vi "Simulation.vi"() -> ()   [LabVIEW 2025]
uses:
  <vilib>/Platform/TimedLoop/XDataNode/timing_clust.ctl
  <vilib>/Platform/TimedLoop/XDataNode/nitl_modes.ctl
  <vilib>/Platform/TimedLoop/XDataNode/wakeup.ctl
  <vilib>/Analysis/5stat.llb/RMS (DBL).vi
  <vilib>/platform/TimedLoop/XDataNode/XDataNode.xnode
  <vilib>/Platform/TimedLoop/XDataNode/XDNodeRunTimeDep.lvlib
  <vilib>/Analysis/NI_AALBase.lvlib
  <vilib>/ptbypt/NI_PtbyPt.lvlib
  <vilib>/Analysis/NI_AALPro.lvlib
panel:
  in  "stop":bool
  out "CLoop":i32
  out "TCP loop":i32
  out "velocity":dbl[](graph)
  out "rms error":dbl format="%0.2f"
  out "TCP":errorcluster
  out "Error":string
  out "Done 2":bool caption="TCP Done"
  out "Path":dbl[](graph)
  out "Output":dbl[](graph)
  out "Error":dbl[](graph)
  out "限制上限":bool
  out "Delay":i32
  out "Done":bool caption="Run Done"
  in  "停止":bool
  in  "開始執行":bool
  out "data length":i32
  out "pdl":i32
  out "Total time":i32
  out "Ts":dbl=0.001
  in  "初始化":bool
  # "資料儲存區"
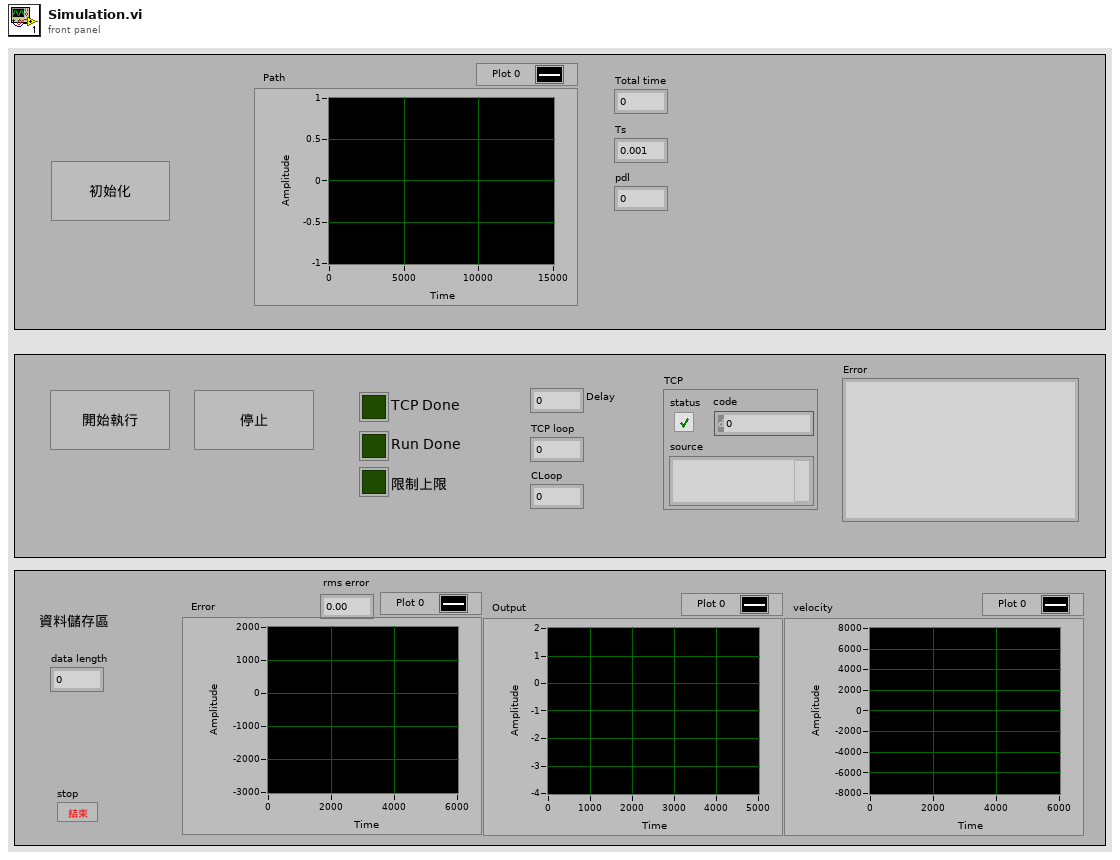
[diagram p1: front panel]
types:
  T1 = typedef "XDNodeRunTimeDep.lvlib/timing_clust.ctl" = cluster{"Expected End [f-1]":u64, "Actual End [f-1]":u64, "Finished Late? [f-1]":bool, "Expected End [i-1]":u64, "Actual End [i-1]":u64, "Finished Late? [i-1]":bool, "Expected Start [i]":u64, "Actual Start [i]":u64, "Expected Start [f]":u64, "Actual Start [f]":u64, "Source Name":string, "Structure Name":string, "Period":i64, "Deadline":i64, "Offset":i64, "Start":i64, "Priority":i32, "Timeout":i32, "Mode":T2, "Wakeup Reason":T3, "Error":errorcluster, "Source Type":string, "Secondary Source Type":string, "Global End Time":u64, "Global Start Time":u64, "Frame Duration":u64, "Iteration Duration":u64, "Assigned CPU":i32, "I/O Scan Engine Mode":u32}
  T2 = typedef "XDNodeRunTimeDep.lvlib/nitl_modes.ctl" = enum32{"No Change", "Process missed periods, maintain original phase", "Discard missed periods, maintain original phase", "Process missed periods, ignore original phase", "Discard missed periods, ignore original phase"}
  T3 = typedef "XDNodeRunTimeDep.lvlib/wakeup.ctl" = enum32{"Normal", "Aborted", "Asynchronous wakeup", "Timing source error", "Timed loop error", "Timeout"}
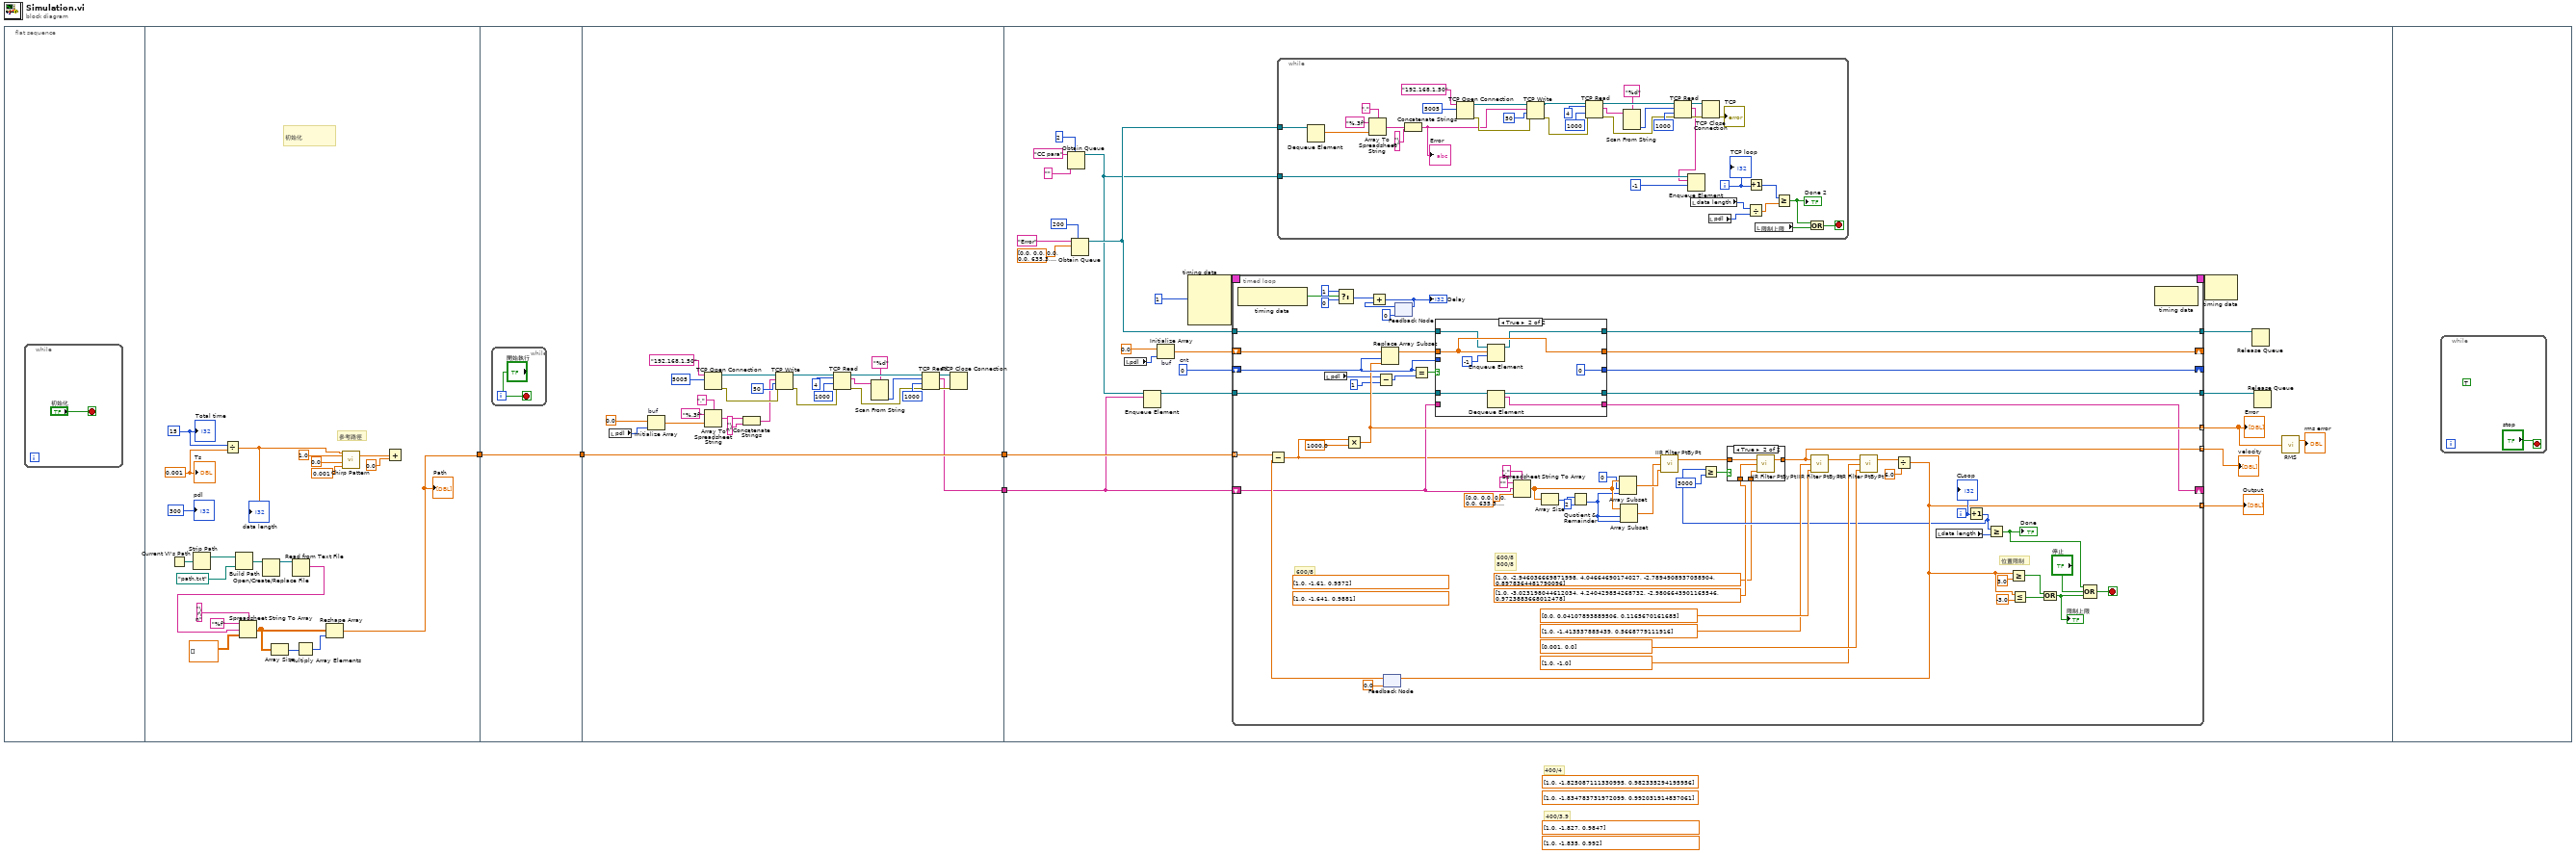
[diagram p0: block diagram]
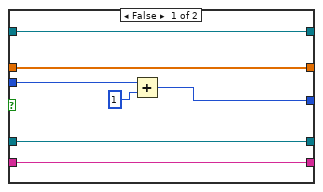
[diagram p3: hidden frame]
diagram:
  (unwired) dbl[] [1.0, -1.835, 0.992] ("Numerator")
  (unwired) dbl[] [1.0, -1.827, 0.9847] ("Numerator")
  (unwired) dbl[] [1.0, -1.834783731972099, 0.992031914837061] ("Numerator")
  (unwired) dbl[] [1.0, -1.825087111330995, 0.982335294195956] ("Numerator")
  # "400/3.9"
  # "400/4"
  n1 = flat-sequence {
    tunnel: [w6] -> w4
    tunnel: [w28] -> w3
    tunnel: w4 -> [w28]
    tunnel: w3 -> [w56]
    tunnel: [w56] -> w2
    tunnel: [w33] -> w1
    tunnel: w2 -> [w77]
    tunnel: w1 -> [w62]
    frame #0 {
      n2 = while {
        stop <- "初始化" stop-if-true
      }
    }
    frame #1 {
      w25 = 15
      w26 = 0.001
      # "參考路徑"
      # "初始化"
      n3 = Current VI's Path() -> (path=w18:path)
      n4 = Strip Path(path=w18) -> (stripped path=w17:path)  [unwired: 1 out]
      n5 = Divide(x=w25, y=w26) -> (x/y=w21:dbl)
      "data length" <- w21
      n6 = Build Path(base path=w17, name or relative path=path "path.txt") -> (appended path=w15:path)
      n7 = Open/Create/Replace File(file path (use dialog)=w15) -> (refnum out=w14:refnum<file>)  [unwired: 5 in, 2 out]
      n8 = Read from Text File(file (use dialog)=w14) -> (text=w11:string)  [unwired: 3 in, 3 out]
      n9 = Spreadsheet String To Array(delimiter (Tab)="\r\n", format string="%f", spreadsheet string=w11, array type (2D Dbl)=dbl[][] []) -> (array=w9:dbl[][])
      n10 = Array Size(array=w9) -> (size(s)=w8:i32[])
      n11 = Multiply Array Elements(1:w8) -> (0:w7:i32)
      n12 = Reshape Array(w9, w7) -> (w6:dbl[])
      "Path" <- w6
      n13 = call <vilib>:"Chirp Pattern.vi"("f2"=0.001, "f1"=0.0, "amplitude"=1.0, "samples"=w21) -> ("Chirp Pattern"=w20:dbl[])  [unwired: 1 out]
      n14 = Add(x=w20, y=0.0) -> ()  [unwired: 1 out]
      "Ts" <- w26
      "Total time" <- w25
      "pdl" <- 300
    }
    frame #2 {
      n15 = while {
        stop <- "開始執行" stop-if-true
      }
    }
    frame #3 {
      n16 = local read "pdl"() -> (w51:i32)
      n17 = Initialize Array "buf"(0.0 ("element"), w51) -> (w52:dbl[])
      n18 = TCP Open Connection(address="192.168.1.50", remote port or service name=u16 5005) -> (connection ID=w48:refnum<k5>, error out=w37:errorcluster)  [unwired: 3 in]
      n19 = Array To Spreadsheet String(delimiter (Tab)=",", array=w52, 3:"%.3f" ("format string")) -> (spreadsheet string=w32:string)
      n20 = Concatenate Strings(w32, "\n" ("string")) -> (w31:string)
      n21 = TCP Write(connection ID=w48, data in=w31, error in (no error)=w37, 9:50 ("timeout ms (25000)")) -> (connection ID out=w38:refnum<k5>, error out=w36:errorcluster)  [unwired: 1 out]
      n22 = TCP Read(connection ID=w38, bytes to read=4, error in (no error)=w36, 9:1000 ("timeout ms (25000)")) -> (connection ID out=w43:refnum<k5>, data out=w42:string, error out=w39:errorcluster)  [unwired: 1 in]
      n23 = Scan From String(format string="%d", input string=w42) -> (output 1=w41:i32)  [unwired: 3 in, 3 out]
      n24 = TCP Read(connection ID=w43, bytes to read=w41, error in (no error)=w39, 9:1000 ("timeout ms (25000)")) -> (connection ID out=w35:refnum<k5>, data out=w33:string, error out=w34:errorcluster)  [unwired: 1 in]
      n25 = TCP Close Connection(connection ID=w35, error in (no error)=w34) -> ()  [unwired: 1 in, 2 out]
    }
    frame #4 {
      w69 = 0  # cnt
      n26 = Obtain Queue(max queue size (-1, unlimited)=2, name (unnamed)="CC para", element data type="") -> (queue out=w61:refnum<queue>)  [unwired: 2 in, 2 out]
      n27 = Obtain Queue(max queue size (-1, unlimited)=200, name (unnamed)="Error", element data type=dbl[] [0.0, 0.0, 0.0, 0.0, 635.3, -3394.0, 6732.0, -5875.0, 1905.0, 0.0]) -> (queue out=w65:refnum<queue>)  [unwired: 2 in, 2 out]
      n28 = local read "pdl"() -> (w63:i32)
      n29 = Enqueue Element(queue=w61, element=w62) -> (queue out=w60:refnum<queue>)  [unwired: 2 in, 2 out]
      n30 = Initialize Array "buf"(0.0 ("element"), w63) -> (w70:dbl[])
      n31 = node-c288(i64 1 ("Period")) -> (w80:T1)  [unwired: 3 in]
      n32 = timed-loop {
        timing: w80 -> [_]
        timing-out: [_] -> w79
        tunnel: w77 -> [w165] mode=indexing
        tunnel: [w125] -> w76 mode=indexing
        tunnel: [w152] -> w58 mode=indexing
        shift-right: [w156] -> _
        shift-left: w70 -> [w160]
        shift-right: [w155] -> _
        shift-left: w69 -> [w157]
        tunnel: w65 -> [w154]
        tunnel: [w151] -> w67
        tunnel: [w149] -> w66
        tunnel: w60 -> [w150]
        shift-right: [w148] -> _
        shift-left: w62 -> [w140]
        tunnel: [w122] -> w57 mode=indexing
        i -> [w162]
        stop <- w124 stop-if-true
        (unwired) dbl[] [1.0, -1.641, 0.9881] ("Numerator")
        (unwired) dbl[] [1.0, -1.61, 0.9572] ("Numerator")
        # "600/8\n800/8"
        # "600/8"
        # "位置限制"
        n33 = node-c288() -> (w167:bool)  [unwired: 1 in]
        n34 = local read "pdl"() -> (w137:i32)
        n35 = Select(t=1, s=w167, f=0) -> (s? t:f=w166:i32)
        n36 = Subtract(x=w137, y=1) -> (x-y=w138:i32)
        n37 = feedback #1(0.0 ("output y(k)")) -> (w164:dbl)
        n38 = Subtract(x=w165, y=w164) -> (x-y=w135:dbl)
        n39 = Multiply(x=w135, y=1000.0) -> (x*y=w152:dbl)
        n40 = Replace Array Subset(array=w160, new element=w152, index=w157) -> (w158:dbl[])
        n41 = feedback #2(0) -> (w169:i32)
        n42 = Add(x=w166, y=w169) -> (x+y=w170:i32)
        "Delay" <- w170
        n43 = feedback-in #2(w170) -> ()
        n44 = Equal?(x=w157, y=w138) -> (x = y?=w159:bool)
        n45 = case shown="True" w159 {
          tunnel: w158 -> [w189 w197]
          tunnel: w157 -> [w190 _]
          tunnel: [w189 w197] -> w156
          tunnel: [w188 0] -> w155
          tunnel: w154 -> [w187 w196]
          tunnel: [w187 w194] -> w151
          tunnel: w150 -> [w186 w195]
          tunnel: [w186 w193] -> w149
          tunnel: [w185 w192] -> w148
          tunnel: w140 -> [w185 _]
          frame False {
            n46 = Add(x=w190, y=1) -> (x+y=w188:i32)
          }
          frame True {
            n47 = Enqueue Element(queue=w196, element=w197, timeout in ms (-1)=-1) -> (queue out=w194:refnum<queue>)  [unwired: 1 in, 2 out]
            n48 = Dequeue Element(queue=w195) -> (queue out=w193:refnum<queue>, element=w192:string)  [unwired: 2 in, 2 out]
          }
        }
        n49 = Spreadsheet String To Array(delimiter (Tab)=",", format string="", spreadsheet string=w140, array type (2D Dbl)=dbl[] [0.0, 0.0, 0.0, 0.0, 635.3, -3394.0, 6732.0, -5875.0, 1905.0, 0.0]) -> (array=w143:dbl[])
        n50 = Array Size(array=w143) -> (size(s)=w145:i32)
        n51 = Quotient & Remainder(x=w145, y=2) -> (floor(x/y)=w139:i32)  [unwired: 1 out]
        n52 = Array Subset(array=w143, index=0, length=w139) -> (w134:dbl[])
        n53 = Array Subset(array=w143, index=w139, length=w139) -> (w133:dbl[])
        n54 = call <vilib>:"IIR Filter PtByPt.vi"("Forward Coefficients"=w134, "Reverse Coefficients"=w133, "x"=w135) -> ("Filtered x"=w123:dbl)  [unwired: 1 in, 1 out]
        n55 = local read "data length"() -> (w174:i32)
        n56 = Increment(x=w162) -> (x+1=w121:i32)
        n57 = Greater Or Equal?(x=w121, y=3000) -> (x >= y?=w119:bool)
        n58 = case shown="True" w119 {
          tunnel: w123 -> [w180 w184]
          tunnel: [w180 w183] -> w122
          tunnel: dbl[] [1.0, -3.023198044612034, 4.240429854268732, -2.9806643901165546, 0.9723883668012478] ("Numerator") -> [_ w182]
          tunnel: dbl[] [1.0, -2.946036669871998, 4.04664690174027, -2.7894908937058904, 0.8978364481790096] ("Numerator") -> [_ w181]
          frame False {
          }
          frame True {
            n59 = call <vilib>:"IIR Filter PtByPt.vi"("Forward Coefficients"=w181, "Reverse Coefficients"=w182, "x"=w184) -> ("Filtered x"=w183:dbl)  [unwired: 1 in, 1 out]
          }
        }
        n60 = call <vilib>:"IIR Filter PtByPt.vi"("Forward Coefficients"=dbl[] [0.0, 0.04107893889506, 0.1165670161685] ("Numerator"), "Reverse Coefficients"=dbl[] [1.0, -1.413537885439, 0.5668779111916] ("Numerator"), "x"=w122) -> ("Filtered x"=w128:dbl)  [unwired: 1 in, 1 out]
        n61 = call <vilib>:"IIR Filter PtByPt.vi"("Forward Coefficients"=dbl[] [0.001, 0.0] ("Numerator"), "Reverse Coefficients"=dbl[] [1.0, -1.0] ("Numerator"), "x"=w128) -> ("Filtered x"=w127:dbl)  [unwired: 1 in, 1 out]
        n62 = Divide(x=w127, y=6.0) -> (x/y=w125:dbl)
        n63 = feedback-in #1(w125) -> ()
        n64 = Greater Or Equal?(x=w121, y=w174) -> (x >= y?=w173:bool)
        "Done" <- w173
        n65 = Greater Or Equal?(x=w125, y=3.0) -> (x >= y?=w177:bool)
        n66 = Less Or Equal?(x=w125, y=-3.0) -> (x <= y?=w176:bool)
        n67 = Compound Arithmetic op=OR(w177, w176) -> (w126:bool)
        "限制上限" <- w126
        n68 = Compound Arithmetic op=OR(w173, "停止", w126) -> (w124:bool)
        n69 = node-c288() -> ()  [unwired: 1 in, 1 out]
        "CLoop" <- w162
      }
      "Error" <- w58
      "Output" <- w76
      "velocity" <- w57
      n70 = while {
        tunnel: w65 -> [w114]
        tunnel: w61 -> [w107]
        i -> [w109]
        stop <- w81 stop-if-true
        n71 = Dequeue Element(queue=w114) -> (element=w108:dbl[])  [unwired: 2 in, 3 out]
        n72 = Array To Spreadsheet String(delimiter (Tab)=",", array=w108, 3:"%.3f" ("format string")) -> (spreadsheet string=w86:string)
        n73 = Concatenate Strings(w86, "\n" ("string")) -> (w84:string)
        "Error" <- w84
        n74 = TCP Open Connection(address="192.168.1.50", remote port or service name=u16 5005) -> (connection ID=w103:refnum<k5>, error out=w92:errorcluster)  [unwired: 3 in]
        n75 = TCP Write(connection ID=w103, data in=w84, error in (no error)=w92, 9:50 ("timeout ms (25000)")) -> (connection ID out=w93:refnum<k5>, error out=w91:errorcluster)  [unwired: 1 out]
        n76 = TCP Read(connection ID=w93, bytes to read=4, error in (no error)=w91, 9:1000 ("timeout ms (25000)")) -> (connection ID out=w98:refnum<k5>, data out=w97:string, error out=w94:errorcluster)  [unwired: 1 in]
        n77 = Scan From String(format string="%d", input string=w97) -> (output 1=w96:i32)  [unwired: 3 in, 3 out]
        n78 = TCP Read(connection ID=w98, bytes to read=w96, error in (no error)=w94, 9:1000 ("timeout ms (25000)")) -> (connection ID out=w90:refnum<k5>, data out=w88:string, error out=w89:errorcluster)  [unwired: 1 in]
        n79 = Enqueue Element(queue=w107, element=w88, timeout in ms (-1)=-1) -> ()  [unwired: 1 in, 3 out]
        n80 = local read "data length"() -> (w113:i32)
        n81 = TCP Close Connection(connection ID=w90, error in (no error)=w89) -> (error out=→"TCP":errorcluster)  [unwired: 1 in, 1 out]
        n82 = local read "pdl"() -> (w112:i32)
        n83 = Divide(x=w113, y=w112) -> (x/y=w110:dbl)
        n84 = Increment(x=w109) -> (x+1=w111:i32)
        n85 = local read "限制上限"() -> (w83:bool)
        n86 = Greater Or Equal?(x=w111, y=w110) -> (x >= y?=w82:bool)
        "Done 2" <- w82
        n87 = Compound Arithmetic op=OR(w82, w83) -> (w81:bool)
        "TCP loop" <- w109
      }
      n88 = node-c288(w79) -> ()  [unwired: 1 out]
      n89 = Release Queue(queue=w67) -> ()  [unwired: 2 in, 3 out]
      n90 = Release Queue(queue=w66) -> ()  [unwired: 2 in, 3 out]
      n91 = call-poly <vilib>:"RMS.vi"("X"=w58) -> ("rms value"=→"rms error":dbl)  [unwired: 1 out]
    }
    frame #5 {
      n92 = while {
        stop <- "stop" stop-if-true
        (unwired) TRUE ("馬達速度歸零")
      }
    }
  }
